vi "Open-Visa-Ethernet-Connection.vi"(2 "Port":string, 3 "IP":string) -> (0 "error out":errorcluster, 1 "VISA resource name out":refnum<visa-resource-name>)   [LabVIEW 2016]
panel:
  out "VISA resource name 3":refnum<visa-resource-name>
  in  "error in (no error)":errorcluster
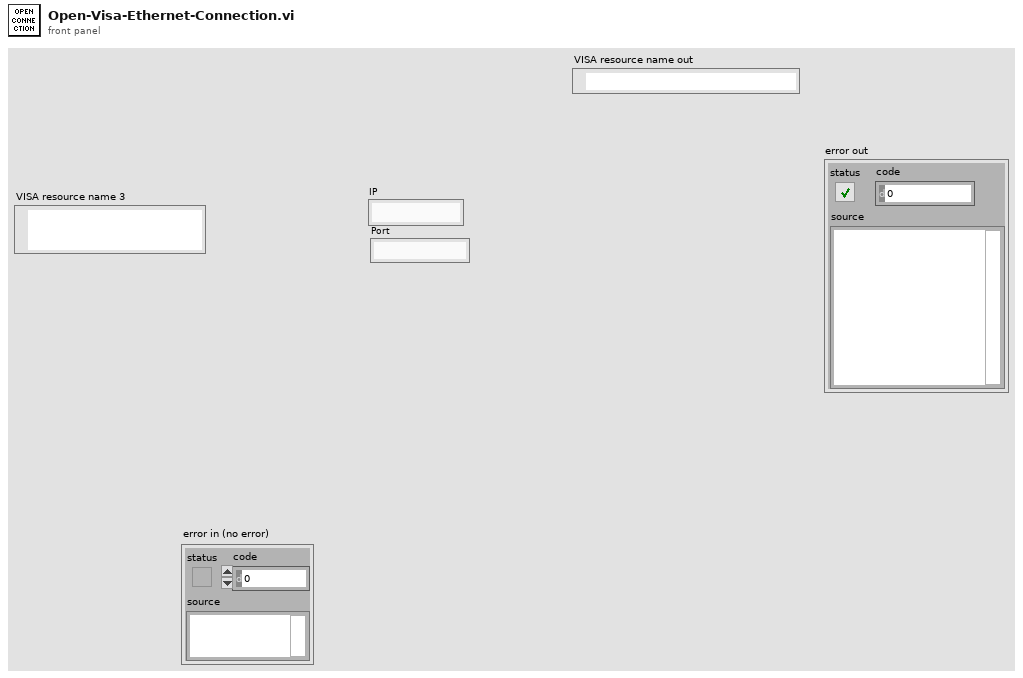
[diagram p1: front panel]
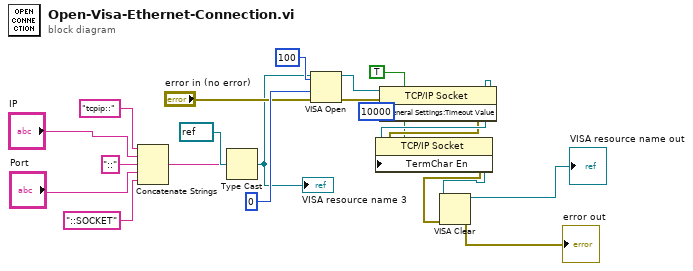
[diagram p0: block diagram]
diagram:
  n1 = Concatenate Strings("tcpip::" ("string"), "IP", "::", "Port", "::SOCKET") -> (w14:string)
  n2 = Type Cast(type=refnum<visa-resource-name> refnum ("VISA resource name"), x=w14) -> (*(type *) &x=w10:refnum<visa-resource-name>)
  "VISA resource name 3" <- w10
  n3 = VISA Open(timeout (0)=u32 100 ("VISA Open timeout (0)"), access mode=u32 0, error in (no error)="error in (no error)", VISA resource name=w10) -> (VISA resource name=w19:refnum<visa-resource-name>, error out=w11:errorcluster)  [unwired: 1 in]
  n4 = property class="TCP/IP Socket"(reference=w19, error in=w11, "General Settings:Timeout Value"=u32 10000) -> (reference out=w18:refnum<visa-resource-name>, error out=w17:errorcluster)
  n5 = property class="TCP/IP Socket"(reference=w18, error in=w17, "TermChar En"=TRUE) -> (reference out=w6:refnum<visa-resource-name>, error out=w5:errorcluster)
  n6 = VISA Clear(VISA resource name=w6, error in (no error)=w5) -> (VISA resource name out=→"VISA resource name out":refnum<visa-resource-name>, error out=→"error out":errorcluster)
